vi "Prueba.vi"() -> ()   [LabVIEW 2013]
panel:
  out "Mucha Calor":bool
  out "Contador":dbl
  out "Temperatura Promedio":dbl
  out "Temperatura Mayor":dbl
  out "Thermometer":i32(slide) scale=0.0..100.0
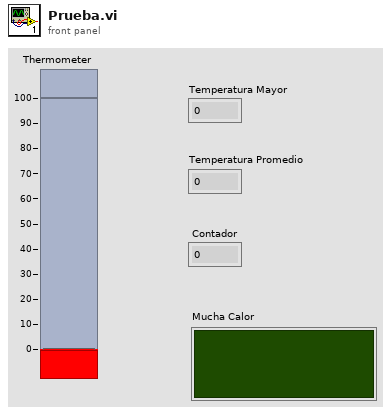
[diagram p1: front panel]
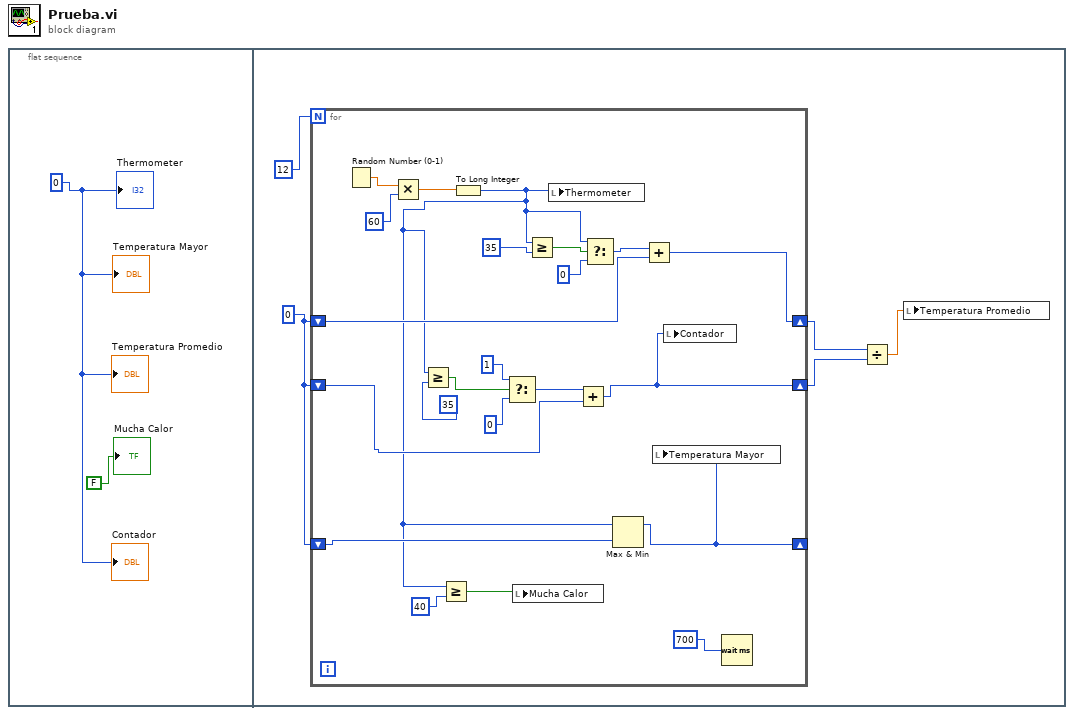
[diagram p0: block diagram]
diagram:
  n1 = flat-sequence {
    frame #0 {
      w2 = 0
      "Thermometer" <- w2
      "Temperatura Promedio" <- w2
      "Contador" <- w2
      "Temperatura Mayor" <- w2
      "Mucha Calor" <- FALSE
    }
    frame #1 {
      w3 = 0
      n2 = for {
        N: 12 -> [_]
        shift-right: [w21] -> w5
        shift-left: w3 -> [w23]
        shift-right: [w15] -> w4
        shift-left: w3 -> [w10]
        shift-right: [w13] -> _
        shift-left: w3 -> [w14]
        n3 = Random Number (0-1)() -> (number: 0 to 1=w29:dbl)
        n4 = Multiply(x=w29, y=60) -> (x*y=w28:dbl)
        n5 = To Long Integer(number=w28) -> (32bit integer=w8:i32)
        n6 = Greater Or Equal?(x=w8, y=35) -> (x >= y?=w18:bool)
        n7 = Greater Or Equal?(x=w8, y=40) -> (x >= y?=w12:bool)
        n8 = Select(t=1, s=w18, f=0) -> (s? t:f=w16:i32)
        n9 = local write "Mucha Calor"(w12) -> ()
        n10 = Greater Or Equal?(x=w8, y=35) -> (x >= y?=w24:bool)
        n11 = local write "Thermometer"(w8) -> ()
        n12 = Add(x=w16, y=w10) -> (x+y=w15:i32)
        n13 = Select(t=w8, s=w24, f=0) -> (s? t:f=w22:i32)
        n14 = Max & Min(x=w8, y=w14) -> (max(x,y)=w13:i32)  [unwired: 1 out]
        n15 = Add(x=w22, y=w23) -> (x+y=w21:i32)
        n16 = local write "Temperatura Mayor"(w13) -> ()
        n17 = local write "Contador"(w15) -> ()
        n18 = Wait (ms)(milliseconds to wait=700) -> ()  [unwired: 1 out]
      }
      n19 = Divide(x=w5, y=w4) -> (x/y=w6:dbl)
      n20 = local write "Temperatura Promedio"(w6) -> ()
    }
  }
